vi "test_read_loop_sync.vi"() -> ()   [LabVIEW 2020, in "UV-VIS_AVANTES.lvclass"]
uses:
  UV-VIS_AVANTES.lvclass
  C:/dev/TRANCON/Classes/GeneralFunctionality/GeneralFunctionality.lvclass
  C:/dev/TRANCON/Classes/Detector/Detector.lvclass
  Config/Config.lvclass
  UV-VIS_AVANTES.lvclass/UV-VIS_AVANTES.ctl
  GeneralFunctionality/GeneralFunctionality.lvclass/GeneralFunctionality.ctl
  Detector.lvclass/Detector.ctl
  Detector.lvclass
  GeneralFunctionality/GeneralFunctionality.lvclass
panel:
  in  "How many":i32=100
  out "String":string
  out "Poll loop":i32
  out "Polled":i32
  out "i":i32
  out "Waveform Graph 2":sgl[](graph)
  out "Waveform Graph":sgl[](graph)
  in  "Path":path=path "C:/Dev/TRANCON/settings/settingsDetector.ini"
  out "error out":errorcluster
  in  "DLL path":path=path "C:/Dev/TRANCON/DLL/avaspec.dll"
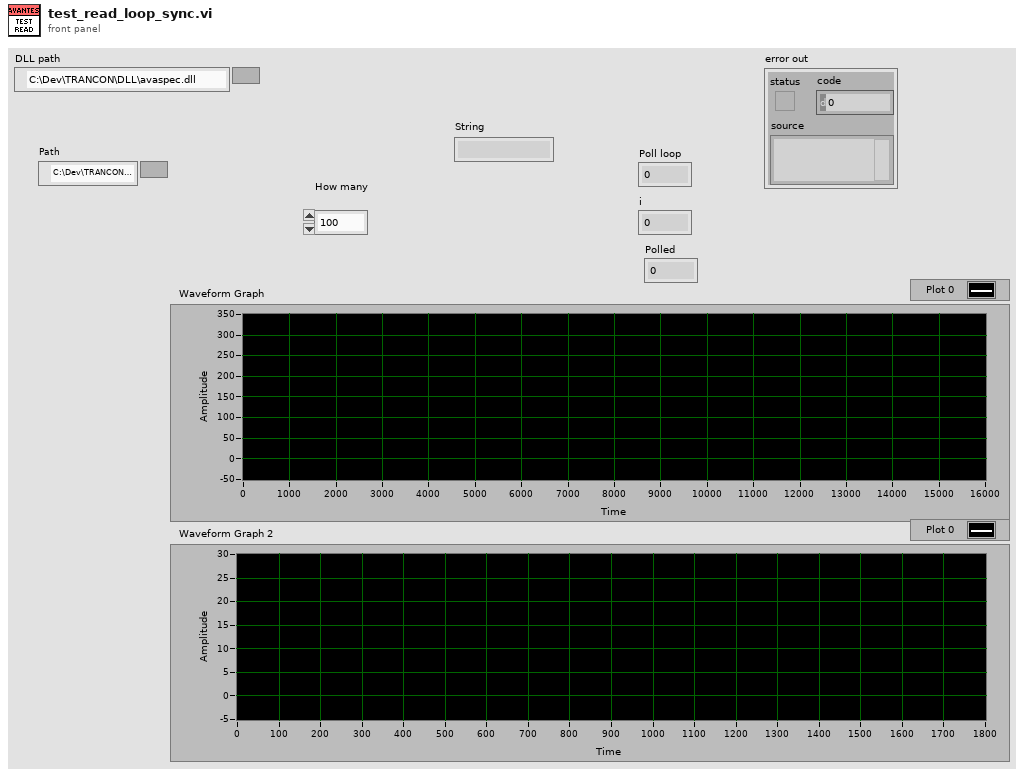
[diagram p1: front panel]
types:
  T1 = typedef "UV-VIS_AVANTES.lvclass/def_parameters.ctl" = cluster{"Len":u16, "ConfigVersion":u16, "UserFriendlyId":u8[], "DetectorType":cluster{"SensorType":u8, "NrPixels":u16, "Fit":sgl[], "NLEnable":u8, "NLCorrect":dbl[], "LowNLCounts":dbl, "HighNLCounts":dbl, "Gain":sgl[], "Reserved":sgl, "Offset":sgl[], "Extern Offset":sgl, "DefectivePixels":u16[]}, "IrradianceType":cluster{"SpectrumCalibrationType":cluster{"SmoothingType":cluster{"m_SmoothPix":u16, "SmoothModel":u8}, "CalInttime":sgl, "CalibConvers":sgl[]}, "CalibrationType":u8, "FiberDiameter":i32}, "SpectrumCalibrationType":cluster{"SmoothingType":cluster{"m_SmoothPix":u16, "SmoothModel":u8}, "CalInttime":sgl, "CalibConvers":sgl[]}, "SpectrumCorrectionType":sgl[], "StandAloneType":cluster{"StandAloneType":u8, "MeasConfigType":cluster{"StartPixel":u16, "StopPixel":u16, "IntegrationTime":sgl, "IntegrationDelay":u32, "NrAverages":u32, "DarkCorrectionType":cluster{"Enable CorDynDark":u8, "ForgetPercentage":u8}, "SmoothingType":cluster{"SmoothPix":u16, "SmoothModel":u8}, "SatDetection":u8, "TriggerType":cluster{"Trigger Mode":u8, "Trigger Source":u8, "Trigger SourceType":u8}, "ControlSettingsType":cluster{"StrobeControl":u16, "LaserDelay":u32, "LaserWidth":u32, "LaserWaveLength":sgl, "StoreToRam":u16}}, "Nmsr":i16}, "DynamicStorageType":cluster{"Nmsr":i32, "Reserved":u8[]}, "TempSensorType":sgl[], "TecControlType":cluster{"Enable":u8, "Setpoint":sgl, "Fit[NR_DAC_POL_COEF]":sgl[]}, "ProcessControlType":cluster{"AnalogLow":sgl[], "AnalogHigh":sgl[], "DigitalLow":sgl[], "DigitalHigh":sgl[]}, "EthernetSettingsType":cluster{"IpAddr":u32, "NetMask":u32, "Gateway":u32, "DhcpEnabled":u8, "TcpPort":u16, "LinkStatus":u8}, "Reserved":u8[]}
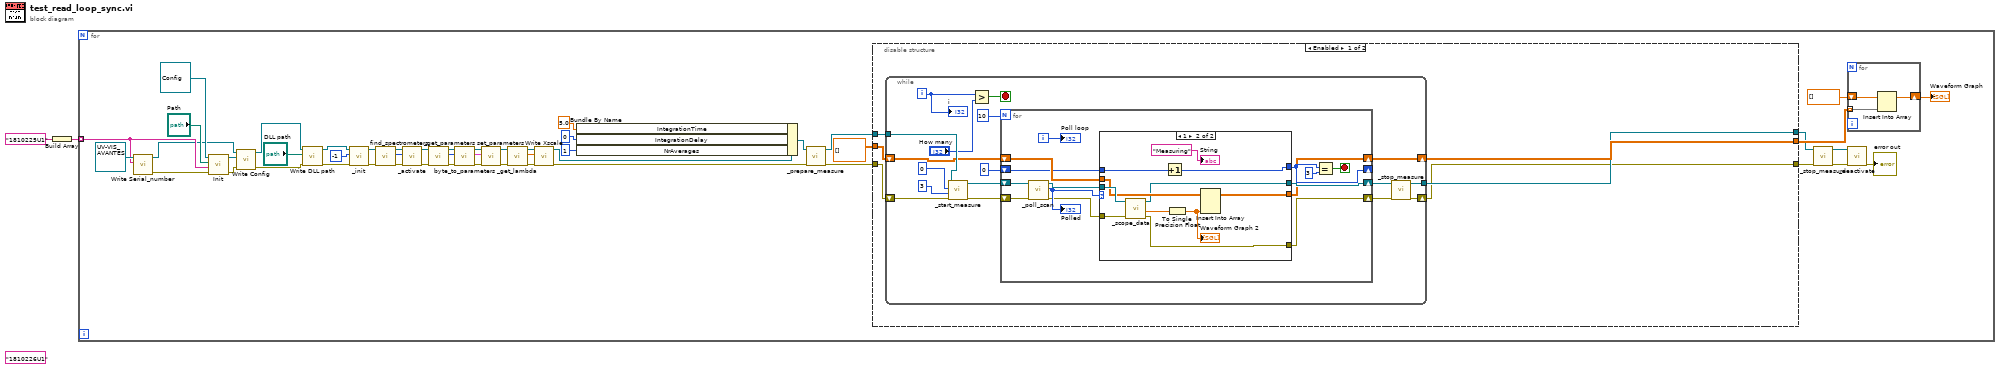
[diagram p0: block diagram]
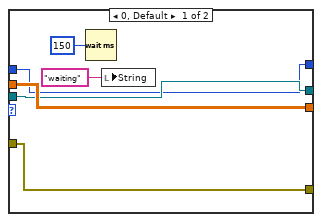
[diagram p2: hidden frame]
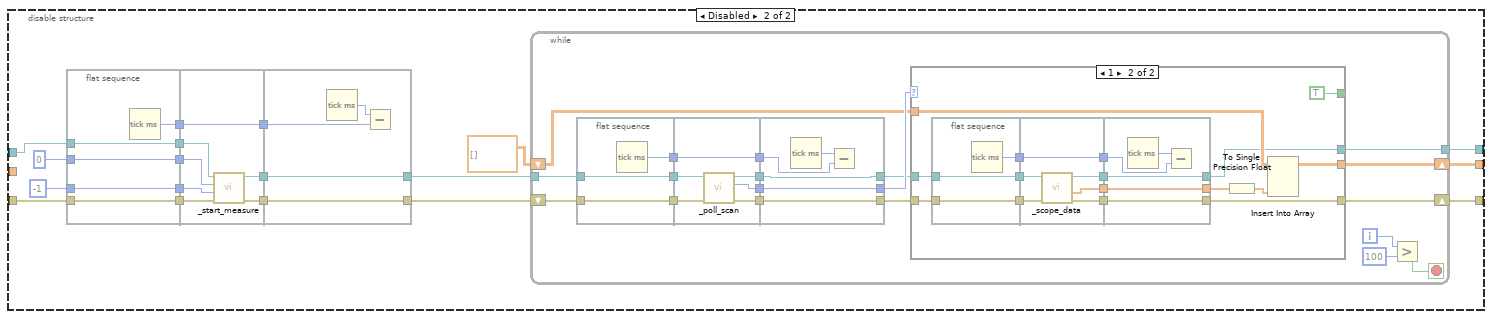
[diagram p3: hidden frame]
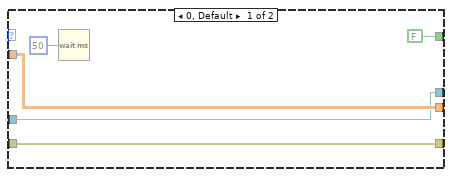
[diagram p4: hidden frame]
diagram:
  (unwired) "1810226U1" ("Serial_number")
  n1 = Build Array("1810225U1" ("Serial_number")) -> (w1:string[])
  n2 = for {
    tunnel: w1 -> [w23] mode=indexing
    n3 = call "Write Serial_number.vi"("Serial_number"=w23, "UV-VIS_AVANTES in"=refnum<class "UV-VIS_AVANTES.lvclass"> refnum ("UV-VIS_AVANTES.lvclass")) -> ("error out"=w22:errorcluster, "UV-VIS_AVANTES out"=w18:refnum<class "UV-VIS_AVANTES.lvclass">)  [unwired: 8 in]
    n4 = call "Init.vi"("error in"=w22, "Name"=w23, "Path"="Path", "Config in"=refnum<class "Config.lvclass"> refnum ("Config.lvclass")) -> ("error out"=w19:errorcluster, "Config out"=w20:refnum<class "Config.lvclass">)  [unwired: 6 in]
    n5 = call "Write Config.vi"("error in (no error)"=w19, "Config.lvclass"=w20, "GeneralFunctionality en entrée"=w18) -> ("error out"=w16:errorcluster, "GeneralFunctionality en sortie"=w17:refnum<class "UV-VIS_AVANTES.lvclass">)  [unwired: 7 in]
    n6 = call "Write DLL path.vi"("error in (no error)"=w16, "DLL path"="DLL path", "Detector in"=w17) -> ("error out"=w32:errorcluster, "Detector out"=w33:refnum<class "UV-VIS_AVANTES.lvclass">)  [unwired: 7 in]
    n7 = call "_init.vi"("error in (no error)"=w32, "a_Port"=i16 -1, "UV-VIS_AVANTES in"=w33) -> ("error out"=w49:errorcluster, "UV-VIS_AVANTES out"=w50:refnum<class "UV-VIS_AVANTES.lvclass">)  [unwired: 6 in, 1 out]
    n8 = call "find_spectrometers.vi"("error in (no error)"=w49, "UV-VIS_AVANTES in"=w50) -> ("error out"=w48:errorcluster, "List Output"=w47:u8[], "UV-VIS_AVANTES out"=w51:refnum<class "UV-VIS_AVANTES.lvclass">)  [unwired: 7 in]
    n9 = call "_activate.vi"("error in (no error)"=w48, "a_pDeviceId IN"=w47, "UV-VIS_AVANTES in"=w51) -> ("error out"=w39:errorcluster, "UV-VIS_AVANTES out"=w40:refnum<class "UV-VIS_AVANTES.lvclass">)  [unwired: 7 in]
    n10 = call "_get_parameters.vi"("error in (no error)"=w39, "UV-VIS_AVANTES in"=w40) -> ("error out"=w46:errorcluster, "DeviceParam"=w45:u8[], "UV-VIS_AVANTES out"=w41:refnum<class "UV-VIS_AVANTES.lvclass">)  [unwired: 7 in]
    n11 = call "byte_to_parameters.vi"("error in (no error)"=w46, "DeviceParam"=w45, "UV-VIS_AVANTES in"=w41) -> ("error out"=w42:errorcluster, "parameters cluster"=w44:T1, "UV-VIS_AVANTES out"=w43:refnum<class "UV-VIS_AVANTES.lvclass">)  [unwired: 6 in]
    n12 = call "set_parameters.vi"("error in (no error)"=w42, "AVS_parameters"=w44, "UV-VIS_AVANTES in"=w43) -> ("error out"=w38:errorcluster, "UV-VIS_AVANTES out"=w37:refnum<class "UV-VIS_AVANTES.lvclass">)  [unwired: 7 in]
    n13 = call "_get_lambda.vi"("error in (no error)"=w38, "UV-VIS_AVANTES in"=w37) -> ("error out"=w34:errorcluster, "a_pWaveLength"=w25:dbl[], "UV-VIS_AVANTES out"=w35:refnum<class "UV-VIS_AVANTES.lvclass">)  [unwired: 7 in]
    n14 = call "Write Xscale.vi"("error in (no error)"=w34, "Xscale"=w25, "Detector en entrée"=w35) -> ("error out"=w11:errorcluster, "Detector en sortie"=w15:refnum<class "UV-VIS_AVANTES.lvclass">)  [unwired: 7 in]
    n15 = Bundle By Name(cluster=w15, "IntegrationTime"=sgl 5.0 ("parameters.StandAloneType.MeasConfigType.IntegrationTime"), "IntegrationDelay"=u32 0 ("parameters.StandAloneType.MeasConfigType.IntegrationDelay"), "NrAverages"=u32 1 ("parameters.StandAloneType.MeasConfigType.NrAverages")) -> (w12:refnum<class "UV-VIS_AVANTES.lvclass">)
    n16 = call "_prepare_measure.vi"("error in (no error)"=w11, "UV-VIS_AVANTES in"=w12) -> ("error out"=w9:errorcluster, "UV-VIS_AVANTES out"=w10:refnum<class "UV-VIS_AVANTES.lvclass">)  [unwired: 7 in, 1 out]
    n17 = disable-structure shown="Enabled" {
      disable-tunnel: w10 -> [w57 w113]
      disable-tunnel: w9 -> [w56 w112]
      disable-tunnel: [w55 w110] -> w8
      disable-tunnel: [w54 w107] -> w5
      disable-tunnel: [w53 w106] -> w4
      disable-tunnel: sgl[][] [] ("Channel I") -> [w52 _]
      frame Enabled {
        n18 = while {
          shift-right: [w61] -> w53
          shift-left: w56 -> [w71]
          tunnel: w57 -> [w72]
          tunnel: [w63] -> w54
          shift-right: [w58] -> w55
          shift-left: w52 -> [w60]
          i -> [w67]
          stop <- w66 stop-if-true
          n19 = call "_start_measure.vi"("error in (no error)"=w71, "a_Nmsr"=i16 3, "a_hWnd"=0, "UV-VIS_AVANTES in"=w72) -> ("error out"=w73:errorcluster, "UV-VIS_AVANTES out"=w74:refnum<class "UV-VIS_AVANTES.lvclass">)  [unwired: 6 in]
          n20 = Greater?(x=w67, y="How many") -> (0:w66:bool)
          n21 = for {
            N: 10 -> [_]
            shift-right: [w86] -> w64
            shift-left: w74 -> [w88]
            shift-right: [w85] -> w62
            shift-left: w73 -> [w87]
            shift-right: [w78] -> _
            shift-left: 0 -> [w79]
            shift-right: [w75] -> w58
            shift-left: w60 -> [w80]
            i -> [w81]
            stop <- w76 stop-if-true
            n22 = call "_poll_scan.vi"("error in (no error)"=w87, "UV-VIS_AVANTES in"=w88) -> ("error out"=w82:errorcluster, "return"=w84:i32, "UV-VIS_AVANTES out"=w83:refnum<class "UV-VIS_AVANTES.lvclass">)  [unwired: 7 in]
            "Polled" <- w84
            n23 = case shown="1" w84 {
              tunnel: w83 -> [w92 w105]
              tunnel: w82 -> [w91 w104]
              tunnel: [w93 w101] -> w75
              tunnel: w80 -> [w93 w102]
              tunnel: [w91 w99] -> w85
              tunnel: [w92 w100] -> w86
              tunnel: w79 -> [w89 w96]
              tunnel: [w89 w95] -> w78
              frame 0, Default {
                n24 = Wait (ms)(milliseconds to wait=u32 150) -> ()  [unwired: 1 out]
                n25 = local write "String"("waiting" ("String")) -> ()
              }
              frame 1 {
                n26 = call "_scope_data.vi"("error in (no error)"=w104, "UV-VIS_AVANTES in"=w105) -> ("error out"=w99:errorcluster, "a_pSpectrum"=w103:dbl[], "UV-VIS_AVANTES out"=w100:refnum<class "UV-VIS_AVANTES.lvclass">)  [unwired: 6 in, 1 out]
                n27 = Increment(x=w96) -> (x+1=w95:i32)
                n28 = To Single Precision Float(number=w103) -> (single precision float=w98:sgl[])
                "Waveform Graph 2" <- w98
                n29 = Insert Into Array(array=w102, new element=w98) -> (w101:sgl[][])  [unwired: 2 in]
                "String" <- "Measuring" ("String")
              }
            }
            n30 = Equal?(x=w78, y=3) -> (x = y?=w76:bool)
            "Poll loop" <- w81
          }
          n31 = call "_stop_measure.vi"("error in (no error)"=w62, "UV-VIS_AVANTES in"=w64) -> ("error out"=w61:errorcluster, "UV-VIS_AVANTES out"=w63:refnum<class "UV-VIS_AVANTES.lvclass">)  [unwired: 8 in]
          "i" <- w67
        }
      }
      frame Disabled {
        n32 = flat-sequence {
          tunnel: i16 -1 ("a_Nmsr") -> [w125]
          tunnel: 0 ("a_hWnd") -> [w126]
          tunnel: w112 -> [w127]
          tunnel: w113 -> [w128]
          tunnel: [w128] -> w123
          tunnel: [w127] -> w122
          tunnel: [w126] -> w121
          tunnel: [w125] -> w120
          tunnel: [w124] -> w119
          tunnel: [w135] -> w118
          tunnel: [w134] -> w117
          tunnel: w123 -> [w133]
          tunnel: w122 -> [w132]
          tunnel: w121 -> [w131]
          tunnel: w120 -> [w130]
          tunnel: w119 -> [w129]
          tunnel: [w129] -> w116
          tunnel: [w138] -> w114
          tunnel: [w139] -> w115
          tunnel: w118 -> [w139]
          tunnel: w117 -> [w138]
          tunnel: w116 -> [w136]
          frame #0 {
            n33 = Tick Count (ms)() -> (millisecond timer value=w124:u32)
          }
          frame #1 {
            n34 = call "_start_measure.vi"("error in (no error)"=w132, "a_Nmsr"=w130, "a_hWnd"=w131, "UV-VIS_AVANTES in"=w133) -> ("error out"=w134:errorcluster, "UV-VIS_AVANTES out"=w135:refnum<class "UV-VIS_AVANTES.lvclass">)  [unwired: 6 in]
          }
          frame #2 {
            n35 = Tick Count (ms)() -> (millisecond timer value=w137:u32)
            n36 = Subtract(x=w137, y=w136) -> ()  [unwired: 1 out]
          }
        }
        n37 = while {
          shift-right: [w155] -> w110
          shift-left: sgl[][] [] ("Channel I") -> [w154]
          shift-right: [w149] -> w106
          shift-left: w114 -> [w152]
          tunnel: w115 -> [w153]
          tunnel: [w148] -> w107
          i -> [w150]
          stop <- w147 stop-if-true
          n38 = flat-sequence {
            tunnel: w152 -> [w160]
            tunnel: w153 -> [w161]
            tunnel: [w161] -> w146
            tunnel: [w160] -> w145
            tunnel: [w159] -> w141
            tunnel: w146 -> [w164]
            tunnel: w145 -> [w163]
            tunnel: [w167] -> w144
            tunnel: [w166] -> w143
            tunnel: [w165] -> w142
            tunnel: w141 -> [w162]
            tunnel: [w162] -> w140
            tunnel: [w170] -> w156
            tunnel: [w171] -> w157
            tunnel: [w172] -> w158
            tunnel: w144 -> [w172]
            tunnel: w143 -> [w171]
            tunnel: w142 -> [w170]
            tunnel: w140 -> [w168]
            frame #0 {
              n39 = Tick Count (ms)() -> (millisecond timer value=w159:u32)
            }
            frame #1 {
              n40 = call "_poll_scan.vi"("error in (no error)"=w163, "UV-VIS_AVANTES in"=w164) -> ("error out"=w165:errorcluster, "return"=w167:i32, "UV-VIS_AVANTES out"=w166:refnum<class "UV-VIS_AVANTES.lvclass">)  [unwired: 7 in]
            }
            frame #2 {
              n41 = Tick Count (ms)() -> (millisecond timer value=w169:u32)
              n42 = Subtract(x=w169, y=w168) -> ()  [unwired: 1 out]
            }
          }
          n43 = case shown="1" w158 {
            tunnel: w157 -> [w174 w193]
            tunnel: w156 -> [w173 w192]
            tunnel: [w176 w189] -> w155
            tunnel: w154 -> [w176 w190]
            tunnel: [FALSE TRUE] -> _
            tunnel: [w173 w186] -> w149
            tunnel: [w174 w187] -> w148
            frame 0, Default {
              n44 = Wait (ms)(milliseconds to wait=u32 50) -> ()  [unwired: 1 out]
            }
            frame 1 {
              n45 = flat-sequence {
                tunnel: w192 -> [w195]
                tunnel: w193 -> [w196]
                tunnel: [w196] -> w184
                tunnel: [w195] -> w183
                tunnel: [w194] -> w178
                tunnel: w184 -> [w202]
                tunnel: w183 -> [w201]
                tunnel: [w200] -> w182
                tunnel: [w199] -> w181
                tunnel: [w198] -> w180
                tunnel: [w197] -> w179
                tunnel: w178 -> [w197]
                tunnel: [w205] -> w186
                tunnel: [w206] -> w187
                tunnel: [w207] -> w191
                tunnel: w182 -> [w207]
                tunnel: w181 -> [w206]
                tunnel: w180 -> [w205]
                tunnel: w179 -> [w203]
                frame #0 {
                  n46 = Tick Count (ms)() -> (millisecond timer value=w194:u32)
                }
                frame #1 {
                  n47 = call "_scope_data.vi"("error in (no error)"=w201, "UV-VIS_AVANTES in"=w202) -> ("error out"=w198:errorcluster, "a_pSpectrum"=w200:dbl[], "UV-VIS_AVANTES out"=w199:refnum<class "UV-VIS_AVANTES.lvclass">)  [unwired: 6 in, 1 out]
                }
                frame #2 {
                  n48 = Tick Count (ms)() -> (millisecond timer value=w204:u32)
                  n49 = Subtract(x=w204, y=w203) -> ()  [unwired: 1 out]
                }
              }
              n50 = To Single Precision Float(number=w191) -> (single precision float=w185:sgl[])
              n51 = Insert Into Array(array=w190, new element=w185) -> (w189:sgl[][])  [unwired: 2 in]
            }
          }
          n52 = Greater?(x=w150, y=100) -> (0:w147:bool)
        }
      }
    }
    n53 = call "_stop_measure.vi"("error in (no error)"=w4, "UV-VIS_AVANTES in"=w5) -> ("error out"=w7:errorcluster, "UV-VIS_AVANTES out"=w6:refnum<class "UV-VIS_AVANTES.lvclass">)  [unwired: 8 in]
    n54 = for {
      shift-right: [w209] -> w13
      shift-left: sgl[] [] ("Channel I") -> [w210]
      tunnel: w8 -> [w208] mode=indexing
      n55 = Insert Into Array(array=w210, new element=w208) -> (w209:sgl[])  [unwired: 1 in]
    }
    "Waveform Graph" <- w13
    n56 = call "_deactivate.vi"("error in (no error)"=w7, "UV-VIS_AVANTES in"=w6) -> ("error out"=→"error out":errorcluster)  [unwired: 8 in, 1 out]
  }
